vi "Streaming - Write Custom Cluster Buffer.vi"() -> ()   [LabVIEW 2020]
uses:
  Nominal Client/Nominal Client.lvclass/Nominal Client.ctl
  e517c7b4-8564-4c59-8860-8935379f7707.vi
  Nominal Client/private_data.set.vi
  <vilib>/Utility/file.llb/Application Directory.vi
  <vilib>/Utility/error.llb/Error Cluster From Error Code.vi
  submodules/reqwest-labview/lv-src/reqwest/create.vi
  stream_custom_cluster/to json.vi
  Nominal Client/http.post.vi
  Nominal Client/Nominal Client.lvclass
  <vilib>/addons/_JKI.lib/REST Client/classes/REST Client/REST Client.lvclass
  nominal types/workspace/workspace.lvclass
  submodules/reqwest-labview/lv-src/reqwest/reqwest.lvclass
  stream_custom_cluster/stream_custom_cluster.lvclass
panel:
  out "Consumer Stopped":bool
  in  "API Token (string or path)":string
  in  "Data Source RID":string
  in  "Stop":bool
  in  "Data Cluster":T1 {"asdfHorizontal Pointer Slide" scale=0.0..10.0}
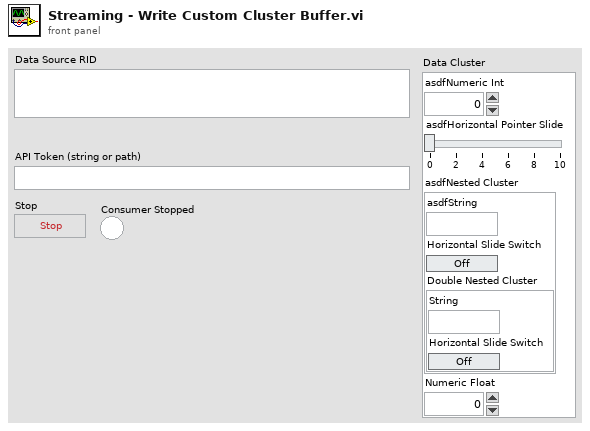
[diagram p1: front panel]
types:
  T1 = cluster{"asdfNumeric Int":i32, "asdfHorizontal Pointer Slide":dbl, "asdfNested Cluster":cluster{"asdfString":string, "Horizontal Slide Switch":bool, "Double Nested Cluster":cluster{"String":string, "Horizontal Slide Switch":bool}}, "Numeric Float":dbl}
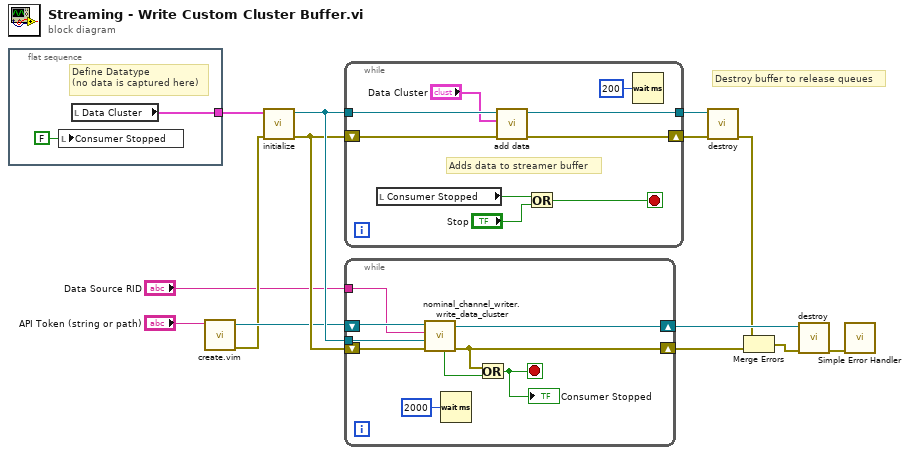
[diagram p0: block diagram]
diagram:
  # "Destroy buffer to release queues"
  n1 = flat-sequence {
    tunnel: [w16] -> w10
    frame #0 {
      # "Define Datatype\n(no data is captured here)"
      n2 = local write "Consumer Stopped"(FALSE ("Consumer Stopped")) -> ()
      n3 = local read "Data Cluster"() -> (w16:T1)
    }
  }
  n4 = call "create.vim"("API Token (string or path)"="API Token (string or path)") -> ("error out"=w8:errorcluster, "Nominal Client"=w9:refnum<class "Nominal Client.lvclass">)  [unwired: 9 in]
  n5 = call "initialize.vi"("error in"=w8, "Data Cluster"=w10) -> ("error out"=w12:errorcluster, "stream custom cluster"=w13:refnum<class "stream_custom_cluster.lvclass">)  [unwired: 8 in]
  n6 = while {
    tunnel: [w24] -> w14
    tunnel: w13 -> [w25]
    shift-right: [w21] -> w11
    shift-left: w12 -> [w22]
    stop <- w17 stop-if-true
    # "Adds data to streamer buffer"
    n7 = local read "Consumer Stopped"() -> (w19:bool)
    n8 = call "add data.vi"("error in"=w22, "Data Cluster"="Data Cluster", "stream custom cluster in"=w25) -> ("error out"=w21:errorcluster, "stream custom cluster out"=w24:refnum<class "stream_custom_cluster.lvclass">)  [unwired: 7 in]
    n9 = Or(x=w19, y="Stop") -> (x .or. y?=w17:bool)
    n10 = Wait (ms)(milliseconds to wait=u32 200) -> ()  [unwired: 1 out]
  }
  n11 = while {
    tunnel: w13 -> [w33]
    shift-right: [w30] -> w7
    shift-left: w9 -> [w31]
    tunnel: "Data Source RID" -> [w29]
    shift-right: [w28] -> w3
    shift-left: w12 -> [w32]
    stop <- w26 stop-if-true
    n12 = call "nominal_channel_writer.write_data_cluster.vi"("error in"=w32, "Custom Cluster Streamer"=w33, "Data Source RID"=w29, "Nominal Client in"=w31) -> ("error out"=w28:errorcluster, "Nominal Client out"=w30:refnum<class "Nominal Client.lvclass">, "Terminated"=w27:bool)  [unwired: 5 in]
    n13 = Wait (ms)(milliseconds to wait=u32 2000) -> ()  [unwired: 1 out]
    n14 = Or(x=w28, y=w27) -> (x .or. y?=w26:bool)
    "Consumer Stopped" <- w26
  }
  n15 = call "destroy.vi"("error in"=w11, "stream custom cluster"=w14) -> ("error out"=w4:errorcluster)  [unwired: 9 in]
  n16 = Merge Errors(w4, w3) -> (w2:errorcluster)
  n17 = call "destroy.vi"("error in"=w2, "Nominal Client"=w7) -> ("error out"=w1:errorcluster)  [unwired: 9 in]
  n18 = call <vilib>:"Simple Error Handler.vi"("error in (no error)"=w1) -> ()  [unwired: 4 in, 5 out]
